vi "SetMode.vi"(8 "Sleep":u32=200, 9 "DoIt":bool=TRUE, 10 "Mode":T1) -> (0 "Sleep":u32)   [LabVIEW 2025]
uses:
  Mode.ctl
  Globals.vi
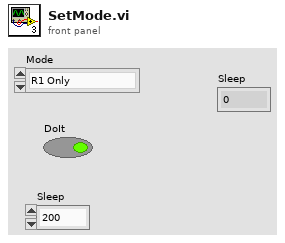
[diagram p1: front panel]
types:
  T1 = typedef "Mode.ctl" = enum16{"R1 Only", "Parallel", "Serial"}
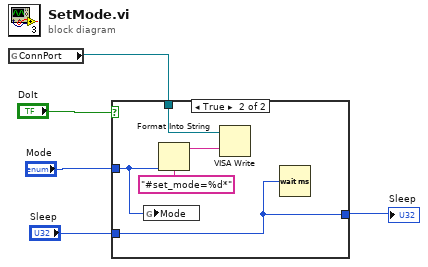
[diagram p0: block diagram]
diagram:
  n1 = global read "Globals.vi" "ConnPort"() -> (w1:refnum<visa-resource-name>)
  n2 = case shown="True" "DoIt" {
    tunnel: "Mode" -> [_ w11]
    tunnel: w1 -> [_ w10]
    tunnel: [w6 w7] -> w4
    tunnel: "Sleep" -> [w6 w7]
    frame False {
    }
    frame True {
      n3 = global write "Globals.vi" "Mode"(w11) -> ()
      n4 = Format Into String(format string="#set_mode=%d*", w11) -> (resulting string=w8:string)  [unwired: 2 in, 1 out]
      n5 = VISA Write(VISA resource name=w10, write buffer=w8) -> ()  [unwired: 1 in, 3 out]
      n6 = Wait (ms)(milliseconds to wait=w7) -> ()  [unwired: 1 out]
    }
  }
  "Sleep" <- w4
